vi "AddDocument.vi"(8 "error in":errorcluster, 10 "FilePath":path, 11 "ProductUnit in":refnum<class "ProductUnit.lvclass">) -> (0 "error out":errorcluster, 2 "Document":refnum<class "Document.lvclass">, 3 "ProductUnit out":refnum<class "ProductUnit.lvclass">)   [LabVIEW 2021, in "ProligentXMLGenerator.lvlib" / "ProductUnit.lvclass"]
doc: "A document defines a link to an external file. This document is uniquely identified by its Identifier.\nThe document also has an optional Name attribute which is meant to contain a human-friendly identifier, and a FileName attribute. The FileName is used to identify the type of document and should contain an extension so that the appropriate application is launched when the user requests to view the document content.\nAn optional Description can also be specified.\n \nDocuments are unique among siblings by their Identifier property. This makes it possible for two different entities (ex: two different product units) to refer to the same document."
uses:
  ProductUnit.lvclass
  Model/Document/Document.lvclass
  ProductUnit.lvclass/ProductUnit.ctl
  <vilib>/Utility/error.llb/Error Cluster From Error Code.vi
  Model/Characteristic/Characteristic.lvclass
  Model/CustomData/CustomData.lvclass
  Base/NonEmptyString_50/NonEmptyString_50.lvclass
  Base/FullName/FullName.lvclass
  Base/Boolean/Boolean.lvclass
  Base/DateTime/DateTime.lvclass
  Base/NonEmptyString_255/NonEmptyString_255.lvclass
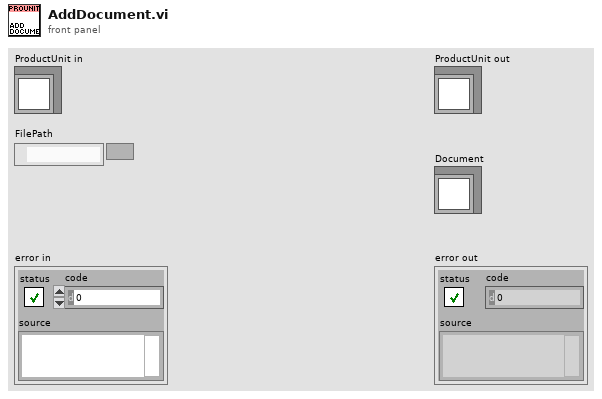
[diagram p1: front panel]
types:
  T1 = typedef "ProligentXMLGenerator.lvlib/ProductUnit.lvclass/Data.ctl" = cluster{"Name":string, "Characteristics":refnum<class "Characteristic.lvclass">[], "Documents":refnum<class "Document.lvclass">[], "CustomData":refnum<class "CustomData.lvclass">, "ProductUnitIdentifier":refnum<class "NonEmptyString_50.lvclass">, "ProductFullName":refnum<class "FullName.lvclass">, "Scrapped":refnum<class "Boolean.lvclass">, "ScrappedTime":refnum<class "DateTime.lvclass">, "CreationTime":refnum<class "DateTime.lvclass">, "ManufacturingTime":refnum<class "DateTime.lvclass">, "ByManufacturer":refnum<class "NonEmptyString_255.lvclass">, "TimeZoneInfoId":string}
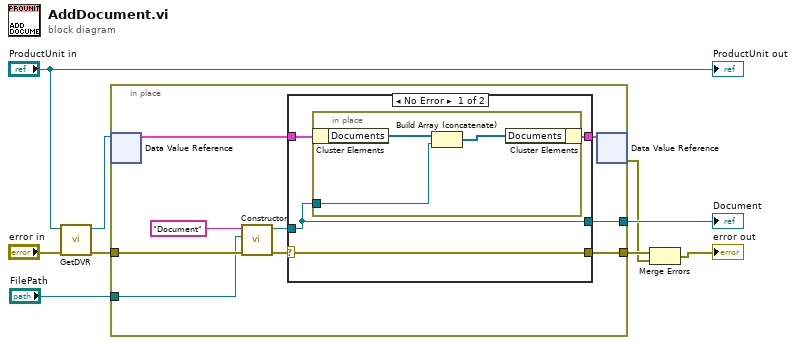
[diagram p0: block diagram]
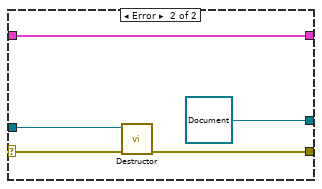
[diagram p2: hidden frame]
diagram:
  n1 = call "GetDVR.vi"("error in"="error in", "ProductUnit in"="ProductUnit in") -> ("error out"=w5:errorcluster, "DVRReference"=w4:refnum<data-value>)  [unwired: 8 in]
  n2 = in-place "In Place Element Structure" {
    in-place-border: [w18] -> w6
    in-place-border: w5 -> [w17]
    in-place-border: [w15] -> w7
    in-place-border: "FilePath" -> [w10]
    n3 = in-place-dvr #1(w4) -> (w12:T1)  [unwired: 1 out]
    n4 = call "Constructor.vi"("error in (no error)"=w17, "FilePath"=w10, "Name"="Document") -> ("error out"=w11:errorcluster, "DocumentType out"=w14:refnum<class "Document.lvclass">)  [unwired: 7 in]
    n5 = case shown="No Error" w11 {
      selector: w11 -> [w22 w29]
      tunnel: [w19 w30] -> w16
      tunnel: [w22 w28] -> w18
      tunnel: w14 -> [w21 w27]
      tunnel: w12 -> [w20 w30]
      tunnel: [w21 refnum<class "Document.lvclass"> refnum ("ProligentResultProcessor:Defect")] -> w15
      frame No Error {
        n6 = in-place "In Place Element Structure" {
          in-place-border: w21 -> [w25]
          n7 = in-place-cluster #2(w20) -> ("Documents"=w24:refnum<class "Document.lvclass">[])
          n8 = Build Array (concatenate)(w24, w25) -> (w23:refnum<class "Document.lvclass">[])
          n9 = in-place-cluster #2("Documents"=w23) -> (w19:T1)
        }
      }
      frame Error {
        n10 = call "Destructor.vi"("error in"=w29, "Document in"=w27) -> ("error out"=w28:errorcluster)  [unwired: 9 in]
      }
    }
    n11 = in-place-dvr #1(w16) -> (w3:errorcluster)  [unwired: 1 out]
  }
  "Document" <- w7
  n12 = Merge Errors(w6, w3) -> (→"error out":errorcluster)
  "ProductUnit out" <- "ProductUnit in"
